vi "BRig_dataLC_Wrong_nRew1_l1.vi"() -> (2 "output_Wrong_nRew1_l1":i32)   [LabVIEW 2014]
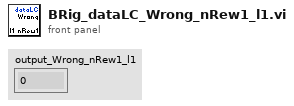
[diagram p1: front panel]
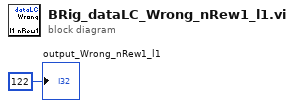
[diagram p0: block diagram]
diagram:
  "output_Wrong_nRew1_l1" <- 122 ("output_iBlock")
